vi "Configure Lbd.vi"   [LabVIEW 2021, in "Ceyear.lvlib"]
doc: "Configures the frequency range for the spectrum analyzer."
uses:
  <instrlib>/Ceyear/Ceyear.lvlib
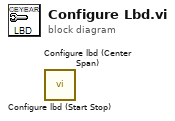
[diagram p0: block diagram]
diagram:
  n1 = call <instrlib>:"Configure lbd (Start Stop).vi"() -> ()  [unwired: 10 in, 2 out]
  n2 = call <instrlib>:"Configure lbd (Center Span).vi"() -> ()  [unwired: 10 in, 2 out]
